vi "Test_numTrip.vi"(3 "error in":errorcluster, 4 "numUninstall":i32, 5 "Break":bool[](array[boolean])) -> (0 "error out":errorcluster, 1 "tripped count":i32, 2 "numTrip":i32)   [LabVIEW 2015]
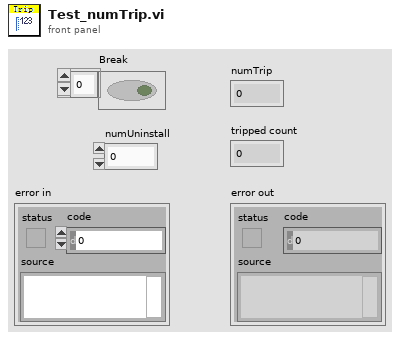
[diagram p1: front panel]
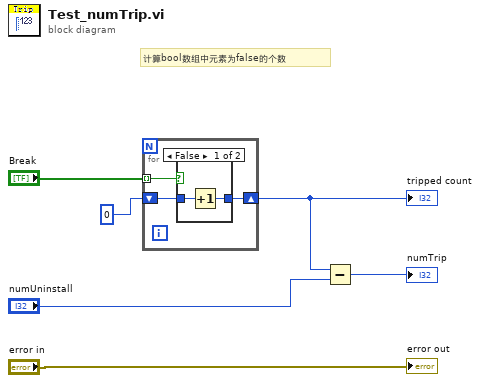
[diagram p0: block diagram]
diagram:
  # "计算bool数组中元素为false的个数"
  n1 = for {
    tunnel: "Break" -> [w9] mode=indexing
    shift-right: [w8] -> w1
    shift-left: 0 -> [w7]
    n2 = case shown="False" w9 {
      tunnel: [w11 w12] -> w8
      tunnel: w7 -> [w10 w12]
      frame False {
        n3 = Increment(x=w10) -> (x+1=w11:i32)
      }
      frame True {
      }
    }
  }
  "tripped count" <- w1
  n4 = Subtract(x=w1, y="numUninstall") -> (x-y=→"numTrip":i32)
  "error out" <- "error in"
